vi "TestRUSHArmControl.vi"() -> ()   [LabVIEW 2012]
panel:
  in  "Setpoint 3":bool
  in  "Setpoint 2":bool
  in  "Setpoint 1":bool
  in  "ClimberHooked":bool
  in  "POTPositions":T1={"Setpoint 1"=1.0, "Setpoint 2"=2.0, "Setpoint 3"=3.0, "Setpoint 4"=4.0, "RotLow"=0.5, "RotHigh"=4.5, "ExtLow"=1.0, "ExtHigh"=4.0}
  in  "ServoPositions":T2={"FlipperLeftUp"=90.0, "FlipperLeftDown"=100.0, "FlipperRightUp"=100.0, "FlipperRightDown"=90.0, "KickerLeftBack"=70.0, "KickerLeftForward"=80.0, "KickerRightBack"=80.0, "KickerRightForward"=70.0}
  in  "WheelBSpd":dbl=0.7
  in  "WheelFSpd":dbl=0.8
  in  "RotPOT":dbl(knob)=2.464558916738698 scale=0.0..5.0
  in  "ExtPOT":dbl(knob)=2.5985477722292334 scale=0.0..5.0
  in  "ExtDeadband":dbl=0.1
  in  "RotDeadband":dbl=0.1
  in  "FlipUp":bool
  in  "YCoord":dbl(slide) scale=-1.0..1.0
  in  "ManualRotate":dbl(slide) scale=-1.0..1.0
  in  "ManualExtend":dbl(slide) scale=-1.0..1.0
  in  "Shoot":bool
  in  "ShootEnableWheels":bool
  in  "VisionTrack":bool
  out "Out Cluster":T3
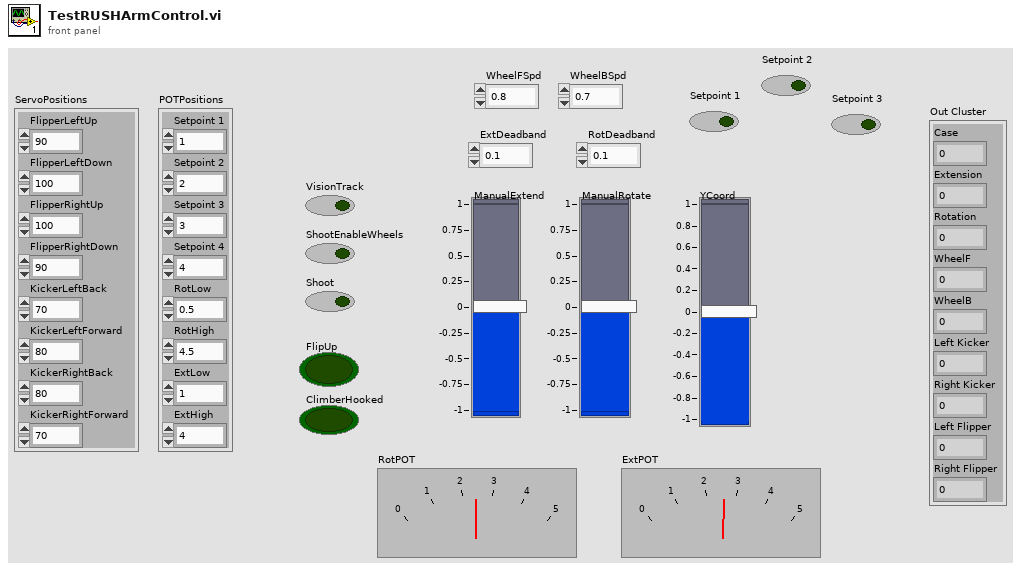
[diagram p1: front panel]
types:
  T1 = cluster{"Setpoint 1":dbl, "Setpoint 2":dbl, "Setpoint 3":dbl, "Setpoint 4":dbl, "RotLow":dbl, "RotHigh":dbl, "ExtLow":dbl, "ExtHigh":dbl}
  T2 = cluster{"FlipperLeftUp":dbl, "FlipperLeftDown":dbl, "FlipperRightUp":dbl, "FlipperRightDown":dbl, "KickerLeftBack":dbl, "KickerLeftForward":dbl, "KickerRightBack":dbl, "KickerRightForward":dbl}
  T3 = cluster{"Case":dbl, "Extension":dbl, "Rotation":dbl, "WheelF":dbl, "WheelB":dbl, "Left Kicker":dbl, "Right Kicker":dbl, "Left Flipper":dbl, "Right Flipper":dbl}
  T4 = cluster{"Case":dbl, "VisionTrack":bool, "ShootEnableWheels":bool, "Shoot":bool, "ManualExtend":dbl, "ManualRotate":dbl, "YCoord":dbl, "FlipUp":bool, "RotDeadband":dbl, "ExtDeadband":dbl, "ExtPOT":dbl, "RotPOT":dbl, "WheelFSpd":dbl, "WheelBSpd":dbl, "ServoPositions":cluster{"FlipperLeftUp":dbl, "FlipperLeftDown":dbl, "FlipperRightUp":dbl, "FlipperRightDown":dbl, "KickerLeftBack":dbl, "KickerLeftForward":dbl, "KickerRightBack":dbl, "KickerRightForward":dbl}, "POTPositions":cluster{"Setpoint 1":dbl, "Setpoint 2":dbl, "Setpoint 3":dbl, "Setpoint 4":dbl, "RotLow":dbl, "RotHigh":dbl, "ExtLow":dbl, "ExtHigh":dbl}, "ClimberHooked":bool}
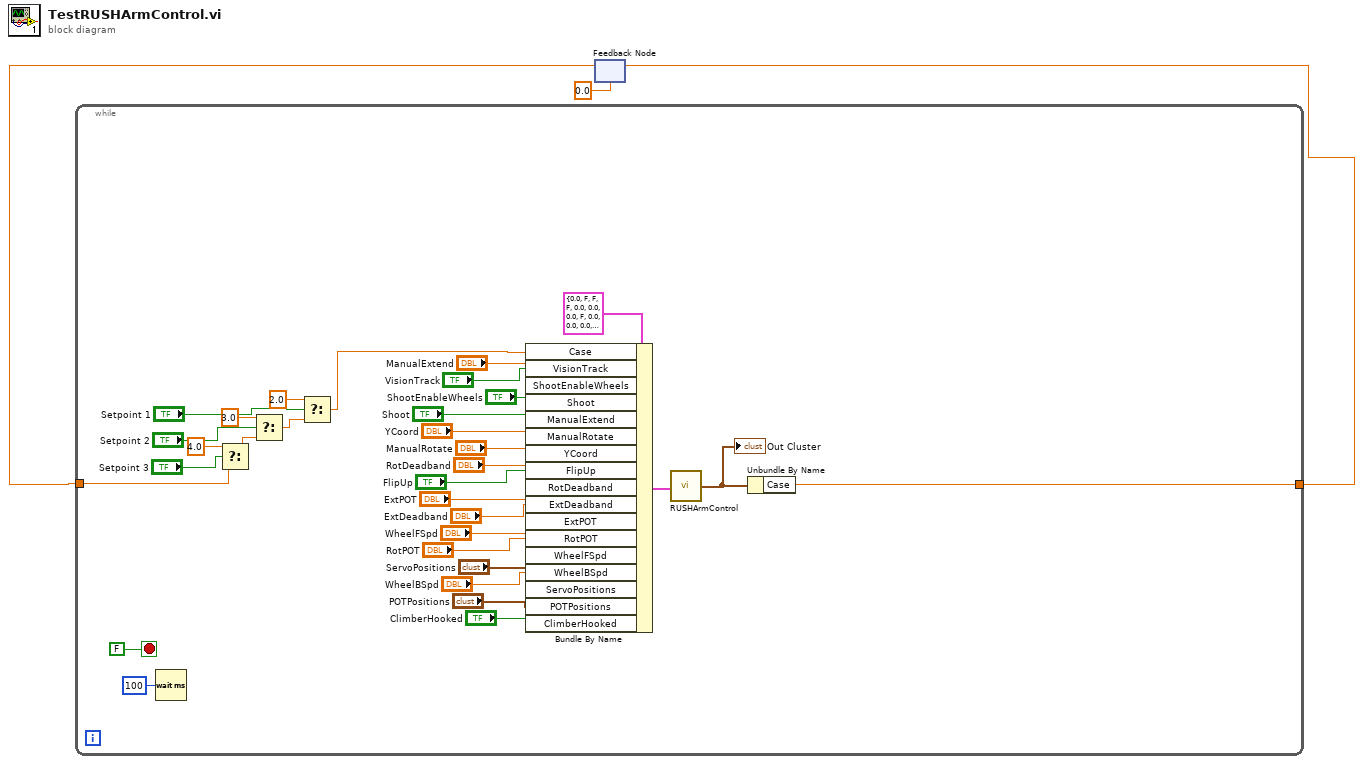
[diagram p0: block diagram]
diagram:
  n1 = feedback #1(0.0 ("Case")) -> (w2:dbl)
  n2 = while {
    tunnel: w2 -> [w8]
    tunnel: [w30] -> w3
    stop <- FALSE stop-if-true
    n3 = Wait (ms)(milliseconds to wait=u32 100) -> ()  [unwired: 1 out]
    n4 = Select(t=4.0, s="Setpoint 3", f=w8) -> (s? t:f=w12:dbl)
    n5 = Select(t=3.0, s="Setpoint 2", f=w12) -> (s? t:f=w13:dbl)
    n6 = Select(t=2.0, s="Setpoint 1", f=w13) -> (s? t:f=w4:dbl)
    n7 = Bundle By Name(cluster=T4 {"Case"=0.0, "VisionTrack"=FALSE, "ShootEnableWheels"=FALSE, "Shoot"=FALSE, "ManualExtend"=0.0, "ManualRotate"=0.0, "YCoord"=0.0, "FlipUp"=FALSE, "RotDeadband"=0.0, "ExtDeadband"=0.0, "ExtPOT"=0.0, "RotPOT"=0.0, "WheelFSpd"=0.0, "WheelBSpd"=0.0, "ServoPositions"={"FlipperLeftUp"=0.0, "FlipperLeftDown"=0.0, "FlipperRightUp"=0.0, "FlipperRightDown"=0.0, "KickerLeftBack"=0.0, "KickerLeftForward"=0.0, "KickerRightBack"=0.0, "KickerRightForward"=0.0}, "POTPositions"={"Setpoint 1"=0.0, "Setpoint 2"=0.0, "Setpoint 3"=0.0, "Setpoint 4"=0.0, "RotLow"=0.0, "RotHigh"=0.0, "ExtLow"=0.0, "ExtHigh"=0.0}, "ClimberHooked"=FALSE} ("In Cluster"), "Case"=w4, "VisionTrack"="VisionTrack", "ShootEnableWheels"="ShootEnableWheels", "Shoot"="Shoot", "ManualExtend"="ManualExtend", "ManualRotate"="ManualRotate", "YCoord"="YCoord", "FlipUp"="FlipUp", "RotDeadband"="RotDeadband", "ExtDeadband"="ExtDeadband", "ExtPOT"="ExtPOT", "RotPOT"="RotPOT", "WheelFSpd"="WheelFSpd", "WheelBSpd"="WheelBSpd", "ServoPositions"="ServoPositions", "POTPositions"="POTPositions", "ClimberHooked"="ClimberHooked") -> (w32:T4)
    n8 = call "RUSHArmControl.vi"("In Cluster"=w32) -> ("Out Cluster"=w31:T3)
    "Out Cluster" <- w31
    n9 = Unbundle By Name(w31) -> ("Case"=w30:dbl)
  }
  n10 = feedback-in #1(w3) -> ()
